vi "Get and Initialize Channel Refs.vi"(8 "error in (no error)":errorcluster, 11 "VS References":T1={"Properties"={"Name"="", "CAN"={"CAN Interface"=enum."CAN1", "Baud Rate"=0, "Diagnostic Protocol"=enum."GMLAN", "Transport Protocol"=enum."ISO TP - Normal Mode", "Transmit ID"=0, "Receive ID"=0, "Transmit Extension"=2, "Receive Extension"=1, "Receive UUDT ID"=0, "Enable Stream"=TRUE, "VW TP Channel ID"=0, "Security"={"Source DLL Path"=path "", "Security Level"=0, "Target DLL Path"=path ""}, "Fill Frame"=FALSE, "Fill Byte"=255, "Termination"=FALSE}, "986x"={"Enable 986x"=FALSE, "RIO Device"=0, "Bitfile"=path ""}, "Reads"=[], "Frames Lookup"=variant(enum16{"GMLAN", "KWP-2000", "UDS"} enum."GMLAN"), "Writes"=[], "DPIDs"=[], "DPID Lookup"=variant(u32 0), "DTC descriptor"={"DTC Byte Length"=2, "Status Byte Length"=1, "Add Data Byte Length"=1, "Byte Order"=enum."Motorola"}}, "Refs"={"Read Data"=[], "Write Data"={"Refs"=[], "Values"=[]}, "Number of DTCs"=0, "DTCs"=[], "Status"=[], "Command Chanels"=[]}} {"Refs"."Command Chanels" format="%.0x"; "Refs"."Status" format="%.0x"; "Refs"."DTCs" format="%.0x"; "Refs"."Number of DTCs" format="%.0x"; "Refs"."Write Data"."Refs"."Data Reference" format="%.0x"; "Refs"."Read Data" format="%.0x"; "Properties"."Writes"."Signals"."Byte Order" items=["Little Endian", "Big Endian"]; "Properties"."Writes"."Signals"."Data Type" items=["Signed", "Unsigned", "IEEE Float"]; "Properties"."CAN"."Fill Byte" format="%.0x"; "Properties"."CAN"."VW TP Channel ID" format="%.0x"; "Properties"."CAN"."Receive UUDT ID" format="%.0x"; "Properties"."CAN"."Receive Extension" format="%.0x"; "Properties"."CAN"."Transmit Extension" format="%.0x"; "Properties"."CAN"."Receive ID" format="%.0x"; "Properties"."CAN"."Transmit ID" format="%.0x"; "Properties"."Reads"."Signals"."Byte Order" items=["Little Endian", "Big Endian"]; "Properties"."Reads"."Signals"."Data Type" items=["Signed", "Unsigned", "IEEE Float"]}) -> (0 "error out":errorcluster, 2 "FPGA Session":u32, 3 "VS Main Configuration":T18={"Properties"={"Name"="", "CAN"={"CAN Interface"=enum."CAN0", "Baud Rate"=0, "Diagnostic Protocol"=enum."GMLAN", "Transport Protocol"=enum."ISO TP - Normal Mode", "Transmit ID"=0, "Receive ID"=0, "Transmit Extension"=0, "Receive Extension"=0, "Receive UUDT ID"=0, "Enable Stream"=TRUE, "VW TP Channel ID"=0, "Security"={"Source DLL Path"=path "", "Security Level"=1, "Target DLL Path"=path ""}, "Fill Frame"=FALSE, "Fill Byte"=255, "Termination"=FALSE}, "986x"={"Enable 986x"=FALSE, "RIO Device"=0, "Bitfile"=path ""}, "Reads"=[], "Frames Lookup"=variant, "Writes"=[], "DPIDs"=[], "DPID Lookup"=variant, "DTC descriptor"={"DTC Byte Length"=2, "Status Byte Length"=1, "Add Data Byte Length"=1, "Byte Order"=enum."Motorola"}}, "ChanRefs"={"ToVS.Reads"={"Name"="", "Write to VS Engine FIFO"=refnum, "Pairs"={"Refs"=[], "Values"=[]}}, "ToVS.DTCs"={"Name"="", "Write to VS Engine FIFO"=refnum, "Pairs"={"Refs"=[], "Values"=[]}}, "ToVS.DTCCount"={"Name"="", "Write to VS Engine FIFO"=refnum, "Pairs"={"Refs"=[], "Values"=[]}}, "ToVS.Status"={"Name"="", "Write to VS Engine FIFO"=refnum, "Pairs"={"Refs"=[], "Values"=[]}}, "FromVS.Writes"={"Name"="", "Read from VS Engine FIFO"=refnum, "Pairs"={"Refs"=[], "Values"=[]}}, "Cmds"={"Name"="", "Write to VS Engine FIFO"=refnum, "Read from VS Engine FIFO"=refnum, "Pairs"={"Chan Refs"=[], "Prev. Values"=[]}}}} {"ChanRefs"."Cmds"."Pairs"."Chan Refs" format="%.0x"; "ChanRefs"."FromVS.Writes"."Pairs"."Refs"."Data Reference" format="%.0x"; "ChanRefs"."ToVS.Status"."Pairs"."Refs" format="%.0x"; "ChanRefs"."ToVS.DTCCount"."Pairs"."Refs" format="%.0x"; "ChanRefs"."ToVS.DTCs"."Pairs"."Refs" format="%.0x"; "ChanRefs"."ToVS.Reads"."Pairs"."Refs" format="%.0x"; "Properties"."Writes"."Signals"."Byte Order" items=["Little Endian", "Big Endian"]; "Properties"."Writes"."Signals"."Data Type" items=["Signed", "Unsigned", "IEEE Float"]; "Properties"."CAN"."Fill Byte" format="%.0x"; "Properties"."CAN"."VW TP Channel ID" format="%.0x"; "Properties"."CAN"."Receive UUDT ID" format="%.0x"; "Properties"."CAN"."Receive Extension" format="%.0x"; "Properties"."CAN"."Transmit Extension" format="%.0x"; "Properties"."CAN"."Receive ID" format="%.0x"; "Properties"."CAN"."Transmit ID" format="%.0x"; "Properties"."Reads"."Signals"."Byte Order" items=["Little Endian", "Big Endian"]; "Properties"."Reads"."Signals"."Data Type" items=["Signed", "Unsigned", "IEEE Float"]})   [LabVIEW 2015, in "Diagnostics Addon Engine.lvlib"]
uses:
  Diagnostics Addon Engine.lvlib
  <vilib>/NI Veristand/Custom Device API/Data Reference.ctl
  <vilib>/NI Veristand/Custom Device API/Custom Device API.lvlib
  <vilib>/NI Veristand/Custom Device API/Block Data Reference.ctl
  Types/VS Data Channels.ctl
  Shared/Types/Protocol.ctl
  Shared/Diagnostics Addon Shared.lvlib
  Shared/Types/CAN.Interface.ctl
  Shared/Types/CAN.ctl
  Types/Main Configuration.ctl
  Shared/Types/Signal.ctl
  Shared/Types/DPID.Rate.ctl
  Shared/Types/DPID.ctl
  Shared/Types/SysDef.Compile.Properties.ctl
  Inline Async API/Inline Async API.lvlib
  Shared/Types/Transport.ctl
  Inline Async API/Controls/ReadWrite Data.ctl
  Inline Async API/Controls/Read From VS Engine.ctl
  Inline Async API/Controls/Write To VS Engine.ctl
  Shared/Types/Security.ctl
  Shared/Types/Frame.Compile.ctl
  Shared/Types/Type.ctl
  Shared/Types/DTCDescriptor.ctl
  Shared/Types/986x.ctl
  Shared/Types/SysDef.Compile.ctl
  Shared/Types/SysDef.Compile.Refs.ctl
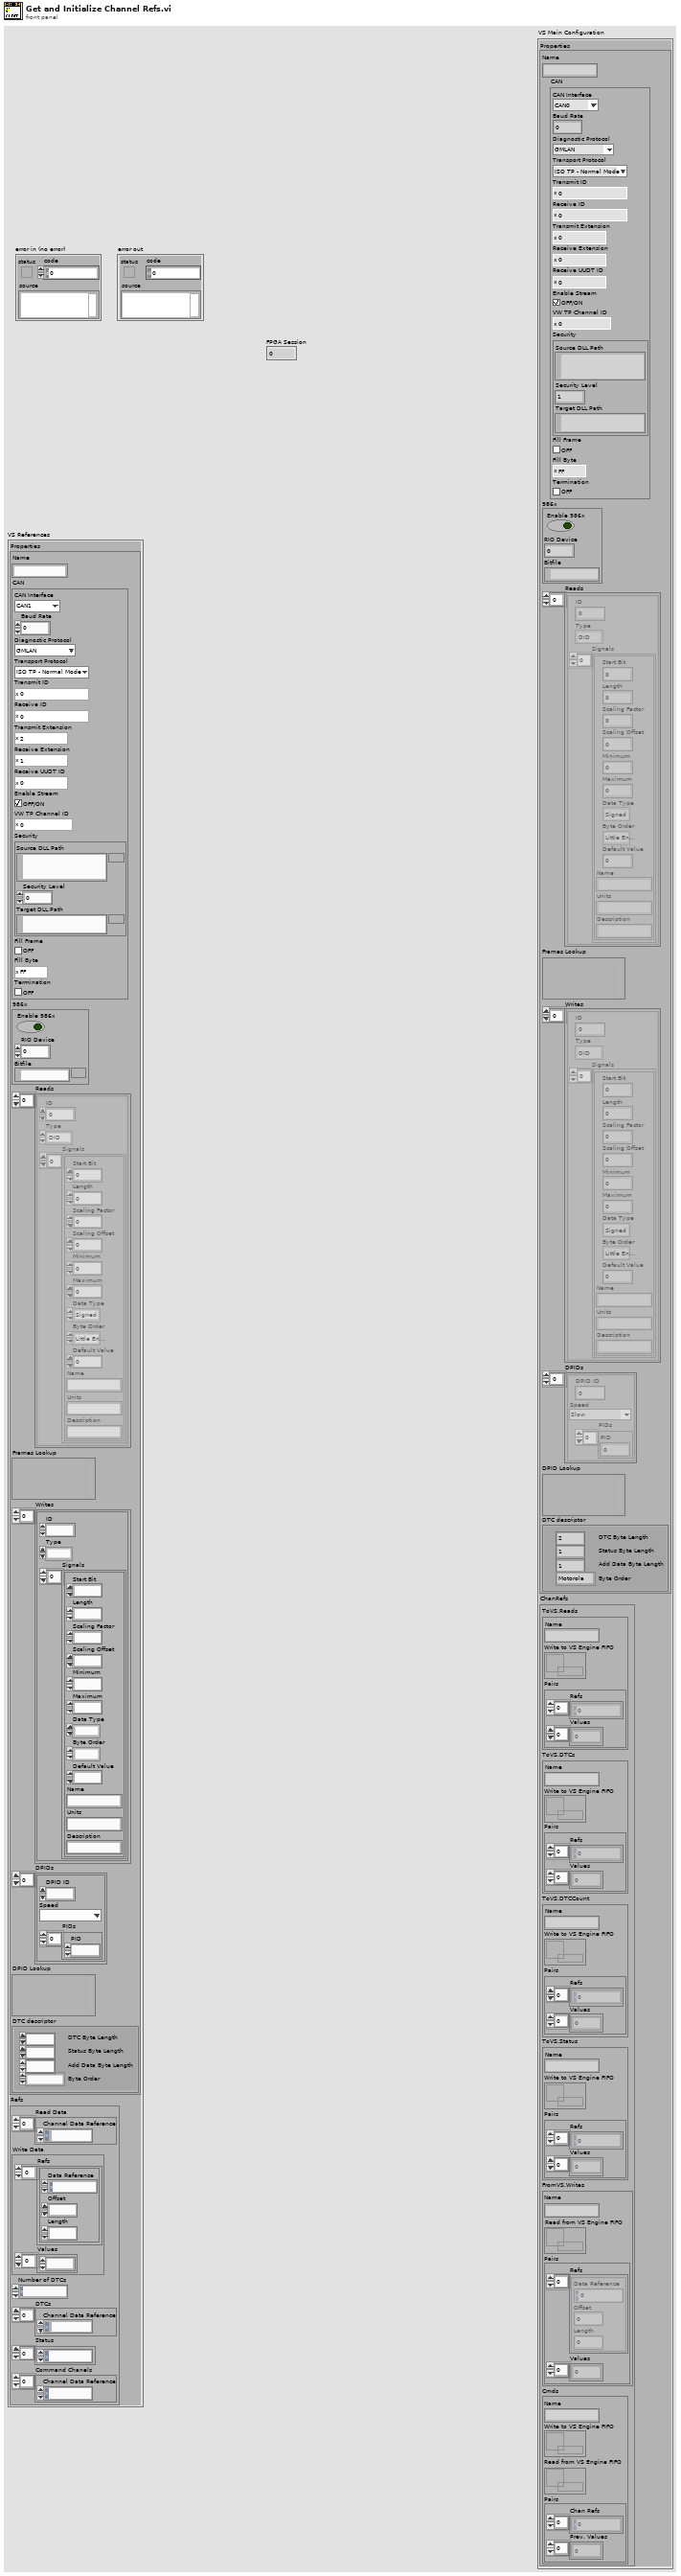
[diagram p1: front panel]
types:
  T1 = typedef "Diagnostics Addon Shared.lvlib/SysDef.Compile.ctl" = cluster{"Properties":T2, "Refs":T15}
  T2 = typedef "Diagnostics Addon Shared.lvlib/SysDef.Compile.Properties.ctl" = cluster{"Name":string, "CAN":T3, "986x":T8, "Reads":T9[], "Frames Lookup":variant, "Writes":T9[], "DPIDs":T12[], "DPID Lookup":variant, "DTC descriptor":T14}
  T3 = typedef "Diagnostics Addon Shared.lvlib/CAN.ctl" = cluster{"CAN Interface":T4, "Baud Rate":u32, "Diagnostic Protocol":T5, "Transport Protocol":T6, "Transmit ID":u32, "Receive ID":u32, "Transmit Extension":u8, "Receive Extension":u8, "Receive UUDT ID":u32, "Enable Stream":bool, "VW TP Channel ID":u32, "Security":T7, "Fill Frame":bool, "Fill Byte":u8, "Termination":bool}
  T4 = typedef "Diagnostics Addon Shared.lvlib/CAN.Interface.ctl" = enum16{"CAN0", "CAN1", "CAN2", "CAN3", "CAN4", "CAN5", "CAN6", "CAN7", "CAN8", "CAN9", "CAN10", "CAN11", "CAN12", "CAN13", "CAN14", "CAN15", "CAN16", "CAN17", "CAN18", "CAN19", "CAN20", "CAN21", "CAN22", "CAN23", "CAN24", "CAN25", "CAN26", "CAN27", "CAN28", "CAN29", "CAN30", "CAN31", "CAN32", "CAN33", "CAN34", "CAN35", "CAN36", "CAN37", "CAN38", "CAN39", "CAN40", "CAN41", "CAN42", "CAN43", "CAN44", "CAN45", "CAN46", "CAN47", "CAN48", "CAN49", "CAN50", "CAN51", "CAN52", "CAN53", "CAN54", "CAN55", "CAN56", "CAN57", "CAN58", "CAN59", "CAN60", "CAN61", "CAN62", "CAN63", "CAN 256 (Virtual)", "CAN 257 (Virtual)"}
  T5 = typedef "Diagnostics Addon Shared.lvlib/Protocol.ctl" = enum16{"GMLAN", "KWP-2000", "UDS"}
  T6 = typedef "Diagnostics Addon Shared.lvlib/Transport.ctl" = enum16{"ISO TP - Normal Mode", "ISO TP - Mixed Mode", "VW TP 2.0", "Diagnostics on IP"}
  T7 = typedef "Diagnostics Addon Shared.lvlib/Security.ctl" = cluster{"Source DLL Path":path, "Security Level":u8, "Target DLL Path":path}
  T8 = typedef "Diagnostics Addon Shared.lvlib/986x.ctl" = cluster{"Enable 986x":bool, "RIO Device":u16, "Bitfile":path}
  T9 = typedef "Diagnostics Addon Shared.lvlib/Frame.Compile.ctl" = cluster{"ID":u32, "Type":T10, "Signals":T11[]}
  T10 = typedef "Diagnostics Addon Shared.lvlib/Type.ctl" = enum16{"DID", "CDID", "PID", "CPID", "Read Memory", "Write Memory", "DTC Control", "IO Cmd", "IO Resp", "Routine Start Cmd", "Routine Start Resp", "Routine Request Cmd", "Routine Request Resp", "Routine Stop Cmd", "Routine Stop Resp"}
  T11 = typedef "Diagnostics Addon Shared.lvlib/Signal.ctl" = cluster{"Start Bit":u8, "Length":u8, "Scaling Factor":dbl, "Scaling Offset":dbl, "Minimum":dbl, "Maximum":dbl, "Data Type":u32, "Byte Order":u32, "Default Value":dbl, "Name":string, "Units":string, "Description":string}
  T12 = typedef "Diagnostics Addon Shared.lvlib/DPID.ctl" = cluster{"DPID ID":u8, "Speed":T13, "PIDs":u16[]}
  T13 = typedef "Diagnostics Addon Shared.lvlib/DPID.Rate.ctl" = enum16{"Slow", "Medium", "Fast"}
  T14 = typedef "Diagnostics Addon Shared.lvlib/DTCDescriptor.ctl" = cluster{"DTC Byte Length":i32, "Status Byte Length":i32, "Add Data Byte Length":i32, "Byte Order":enum16{"Motorola", "Intel"}}
  T15 = typedef "Diagnostics Addon Shared.lvlib/SysDef.Compile.Refs.ctl" = cluster{"Read Data":T16[], "Write Data":cluster{"Refs":T17[], "Values":dbl[]}, "Number of DTCs":T16, "DTCs":T16[], "Status":T16[], "Command Chanels":T16[]}
  T16 = typedef "Custom Device API.lvlib/Data Reference.ctl" = i32
  T17 = typedef "Custom Device API.lvlib/Block Data Reference.ctl" = cluster{"Data Reference":T16, "Offset":u64, "Length":u64}
  T18 = typedef "Diagnostics Addon Engine.lvlib/Main Configuration.ctl" = cluster{"Properties":T2, "ChanRefs":T19}
  T19 = typedef "Diagnostics Addon Engine.lvlib/VS Data Channels.ctl" = cluster{"ToVS.Reads":T20, "ToVS.DTCs":T20, "ToVS.DTCCount":T20, "ToVS.Status":T20, "FromVS.Writes":T21, "Cmds":T22}
  T20 = typedef "Diagnostics Addon Engine.lvlib/Inline Async API.lvlib/Write To VS Engine.ctl" = cluster{"Name":string, "Write to VS Engine FIFO":refnum<k33>, "Pairs":cluster{"Refs":T16[], "Values":dbl[]}}
  T21 = typedef "Diagnostics Addon Engine.lvlib/Inline Async API.lvlib/Read From VS Engine.ctl" = cluster{"Name":string, "Read from VS Engine FIFO":refnum<k33>, "Pairs":cluster{"Refs":T17[], "Values":dbl[]}}
  T22 = typedef "Diagnostics Addon Engine.lvlib/Inline Async API.lvlib/ReadWrite Data.ctl" = cluster{"Name":string, "Write to VS Engine FIFO":refnum<k33>, "Read from VS Engine FIFO":refnum<k33>, "Pairs":cluster{"Chan Refs":T16[], "Prev. Values":dbl[]}}
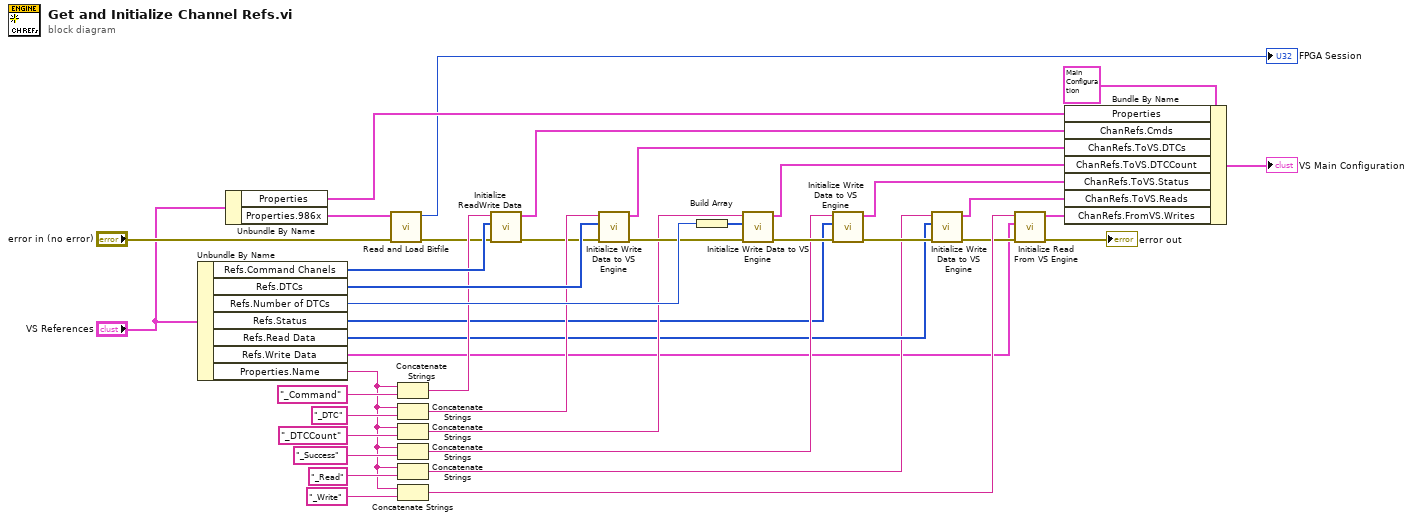
[diagram p0: block diagram]
diagram:
  n1 = Unbundle By Name("VS References") -> ("Refs.Command Chanels"=w39:T16[], "Refs.DTCs"=w31:T16[], "Refs.Number of DTCs"=w35:T16, "Refs.Status"=w15:T16[], "Refs.Read Data"=w7:T16[], "Refs.Write Data"=w3:cluster{"Refs":T17[], "Values":dbl[]}, "Properties.Name"=w5:string)
  n2 = Unbundle By Name("VS References") -> ("Properties"=w17:T2, "Properties.986x"=w18:T8)
  n3 = call "Read and Load Bitfile.vi"("error in (no error)"="error in (no error)", "FPGA Bitfile Settings"=w18) -> ("error out"=w20:errorcluster, "FPGA Session"=→"FPGA Session":u32)  [unwired: 8 in]
  n4 = Concatenate Strings(w5, "_Command" ("string")) -> (w29:string)
  n5 = Concatenate Strings(w5, "_DTC" ("string")) -> (w26:string)
  n6 = Concatenate Strings(w5, "_DTCCount" ("string")) -> (w25:string)
  n7 = Concatenate Strings(w5, "_Success" ("string")) -> (w23:string)
  n8 = Concatenate Strings(w5, "_Read" ("string")) -> (w6:string)
  n9 = Concatenate Strings(w5, "_Write" ("string")) -> (w12:string)
  n10 = call "Initialize ReadWrite Data.vi"("error in (no error)"=w20, "Chan Refs"=w39, "Name"=w29) -> ("error out"=w9:errorcluster, "ReadWrite Data"=w28:T22)  [unwired: 7 in]
  n11 = call "Initialize Write Data to VS Engine.vi"("error in (no error)"=w9, "Hardware Output Refs"=w31, "FIFO Name"=w26) -> ("error out"=w32:errorcluster, "Write to VS Engine"=w27:T20)  [unwired: 7 in]
  n12 = Build Array(w35) -> (w34:T16[])
  n13 = call "Initialize Write Data to VS Engine.vi"("error in (no error)"=w32, "Hardware Output Refs"=w34, "FIFO Name"=w25) -> ("error out"=w33:errorcluster, "Write to VS Engine"=w24:T20)  [unwired: 7 in]
  n14 = call "Initialize Write Data to VS Engine.vi"("error in (no error)"=w33, "Hardware Output Refs"=w15, "FIFO Name"=w23) -> ("error out"=w8:errorcluster, "Write to VS Engine"=w22:T20)  [unwired: 7 in]
  n15 = call "Initialize Write Data to VS Engine.vi"("error in (no error)"=w8, "Hardware Output Refs"=w7, "FIFO Name"=w6) -> ("error out"=w4:errorcluster, "Write to VS Engine"=w1:T20)  [unwired: 7 in]
  n16 = call "Initialize Read From VS Engine.vi"("error in (no error)"=w4, "Pairs"=w3, "FIFO Name"=w12) -> ("error out"=→"error out":errorcluster, "Read from VS Engine"=w11:T21)  [unwired: 7 in]
  n17 = Bundle By Name(cluster=T18 {"Properties"={"Name"="", "CAN"={"CAN Interface"=enum."CAN0", "Baud Rate"=0, "Diagnostic Protocol"=enum."GMLAN", "Transport Protocol"=enum."ISO TP - Normal Mode", "Transmit ID"=0, "Receive ID"=0, "Transmit Extension"=0, "Receive Extension"=0, "Receive UUDT ID"=0, "Enable Stream"=FALSE, "VW TP Channel ID"=0, "Security"={"Source DLL Path"=path "", "Security Level"=0, "Target DLL Path"=path ""}, "Fill Frame"=FALSE, "Fill Byte"=0, "Termination"=FALSE}, "986x"={"Enable 986x"=FALSE, "RIO Device"=0, "Bitfile"=path ""}, "Reads"=[], "Frames Lookup"=variant, "Writes"=[], "DPIDs"=[], "DPID Lookup"=variant, "DTC descriptor"={"DTC Byte Length"=0, "Status Byte Length"=0, "Add Data Byte Length"=0, "Byte Order"=enum."Motorola"}}, "ChanRefs"={"ToVS.Reads"={"Name"="", "Write to VS Engine FIFO"=refnum, "Pairs"={"Refs"=[], "Values"=[]}}, "ToVS.DTCs"={"Name"="", "Write to VS Engine FIFO"=refnum, "Pairs"={"Refs"=[], "Values"=[]}}, "ToVS.DTCCount"={"Name"="", "Write to VS Engine FIFO"=refnum, "Pairs"={"Refs"=[], "Values"=[]}}, "ToVS.Status"={"Name"="", "Write to VS Engine FIFO"=refnum, "Pairs"={"Refs"=[], "Values"=[]}}, "FromVS.Writes"={"Name"="", "Read from VS Engine FIFO"=refnum, "Pairs"={"Refs"=[], "Values"=[]}}, "Cmds"={"Name"="", "Write to VS Engine FIFO"=refnum, "Read from VS Engine FIFO"=refnum, "Pairs"={"Chan Refs"=[], "Prev. Values"=[]}}}}, "Properties"=w17, "ChanRefs.Cmds"=w28, "ChanRefs.ToVS.DTCs"=w27, "ChanRefs.ToVS.DTCCount"=w24, "ChanRefs.ToVS.Status"=w22, "ChanRefs.ToVS.Reads"=w1, "ChanRefs.FromVS.Writes"=w11) -> (→"VS Main Configuration":T18)
